vi "SAVE_CONFIG.vi"(11 "Param_IN":T1={"Init_Onset_Load"=10.0, "Param"={"Clt_Param_L"={"기준값"=90.0, "검출값"=120.0, "Onset_Min"=5.0, "Onset_Max"=10.0, "Peak_Min"=200.0, "Peak_Max"=220.0, "Base"=2000}, "Clt_Param_R"={"기준값"=90.0, "검출값"=120.0, "Onset_Min"=5.0, "Onset_Max"=10.0, "Peak_Min"=200.0, "Peak_Max"=220.0, "Base"=2000}}, "MinPos"=2000, "MaxPos"=230000, "Init_Vel_UP"=5000, "Init_Accel"=10000, "Test_Vel"=1000000, "Test_Acc"=10000000, "Init_Vel_DOWN"=5000, "Load_Warning"=200.0, "Load_Alarm"=300.0}) -> ()   [LabVIEW 2019]
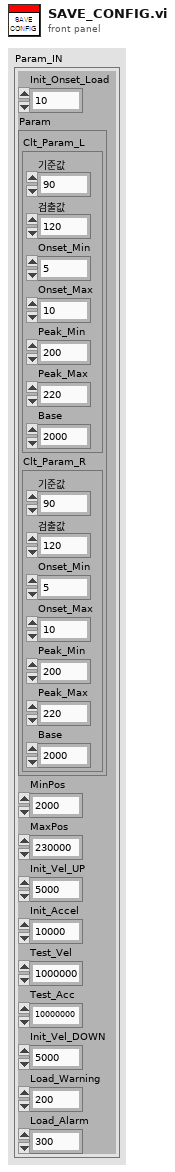
[diagram p1: front panel]
types:
  T1 = cluster{"Init_Onset_Load":sgl, "Param":cluster{"Clt_Param_L":cluster{"기준값":sgl, "검출값":sgl, "Onset_Min":sgl, "Onset_Max":sgl, "Peak_Min":sgl, "Peak_Max":sgl, "Base":i32}, "Clt_Param_R":cluster{"기준값":sgl, "검출값":sgl, "Onset_Min":sgl, "Onset_Max":sgl, "Peak_Min":sgl, "Peak_Max":sgl, "Base":i32}}, "MinPos":i32, "MaxPos":i32, "Init_Vel_UP":i32, "Init_Accel":u32, "Test_Vel":i32, "Test_Acc":u32, "Init_Vel_DOWN":i32, "Load_Warning":sgl, "Load_Alarm":sgl}
  T2 = enum16{"open", "replace", "create", "open or create", "replace or create", "replace or create with confirmation"}
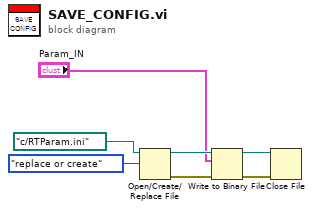
[diagram p0: block diagram]
diagram:
  n1 = Open/Create/Replace File(file path (use dialog)=path "c:/RTParam.ini" ("파일 경로(대화 상자 사용)"), operation (0:open)=T2."replace or create" ("동작(0:open)")) -> (refnum out=w7:refnum<file>, error out=w6:errorcluster)  [unwired: 4 in, 1 out]
  n2 = Write to Binary File(file (use dialog)=w7, data="Param_IN", error in=w6) -> (refnum out=w3:refnum<file>, error out=w2:errorcluster)  [unwired: 3 in, 1 out]
  n3 = Close File(refnum=w3, error in=w2) -> ()  [unwired: 2 out]
